vi "SetdBStep.vi"(8 "错误输入（无错误）":errorcluster, 10 "步进索引值":u16) -> (0 "错误输出":errorcluster)   [LabVIEW 2014]
uses:
  X86Dll/ZXUTConfigMgr.dll
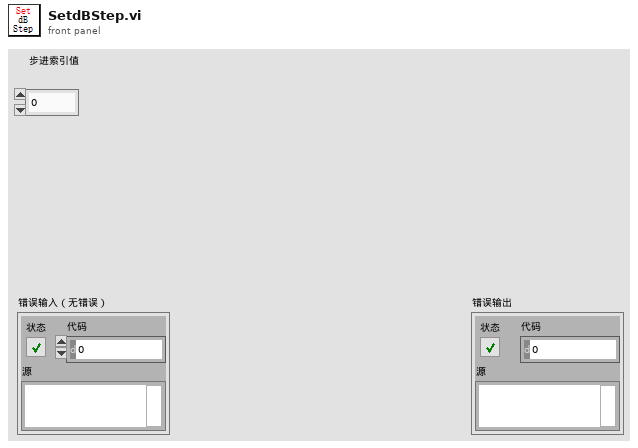
[diagram p1: front panel]
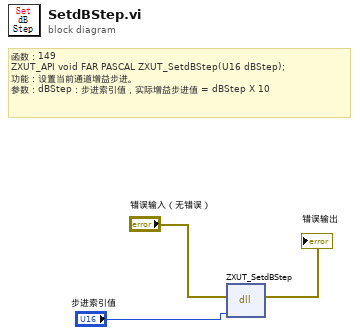
[diagram p0: block diagram]
diagram:
  # "函数：149\nZXUT_API void\tFAR PASCAL ZXUT_SetdBStep(U16 dBStep);\n功能：设置当前通道增益步进。\n参数：dBStep：步进索引值，实际增益步进值 = dBStep X 10"
  n1 = dll-call lib="D:/Software/Utrasonic on-line monitoring/X86Dll/ZXUTConfigMgr.dll" fn="ZXUT_SetdBStep"(error in="错误输入（无错误）", "dBStep"="步进索引值") -> (error out=→"错误输出":errorcluster)  [unwired: 4 in, 1 out]
